vi "Read clEvtReportArray.vi"(8 "error in (no error)":errorcluster, 11 "VisualizeAppBase_class in":refnum<class "VisualizeAppBase_class.lvclass">) -> (0 "error out":errorcluster, 2 "clEvtReportArray":T1 {"Synx" format="%#_4g"}, 3 "VisualizeAppBase_class out":refnum<class "VisualizeAppBase_class.lvclass">)   [LabVIEW 2017, in "Visualization.lvlib" / "VisualizeAppBase_class.lvclass"]
uses:
  VisualizeAppBase_class.lvclass
  Modules/EventPlugins/EventPluginBaseClass/TypeDefs/clEvtReportArray.ctl
  Modules/EventPlugins/EventPluginBaseClass/TypeDefs/clEvtReport.ctl
  VisualizeAppBase_class.lvclass/VisualizeAppBase_class.ctl
  Modules/EventPlugins/EventPluginBaseClass/EventPluginBaseClass.lvclass
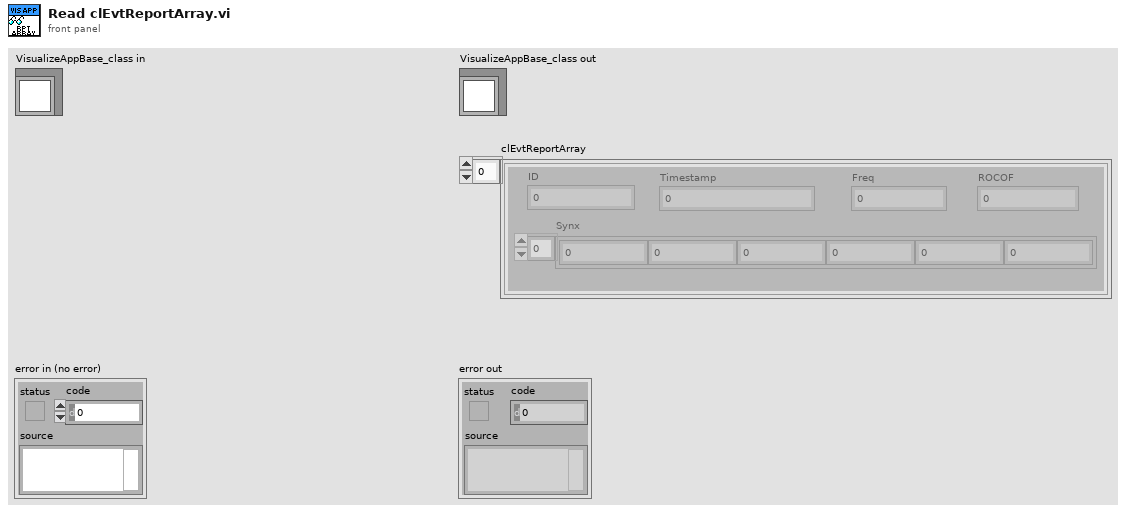
[diagram p1: front panel]
types:
  T1 = typedef "EventPlugins.lvlib/EventPluginBaseClass.lvclass/clEvtReportArray.ctl" = T2[]
  T2 = typedef "EventPlugins.lvlib/EventPluginBaseClass.lvclass/clEvtReport.ctl" = cluster{"Timestamp":dbl, "Synx":cdb[], "Freq":dbl, "ROCOF":dbl, "ID":i16}
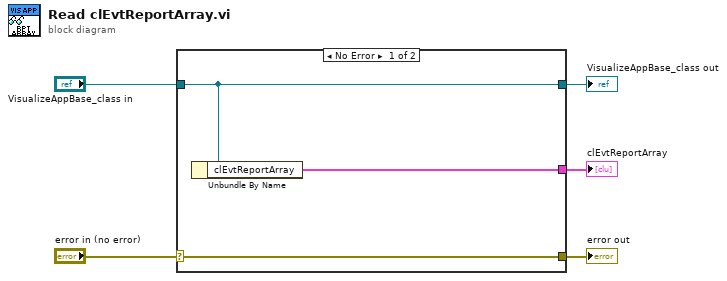
[diagram p0: block diagram]
diagram:
  n1 = case shown="No Error" "error in (no error)" {
    selector: "error in (no error)" -> [w8 w9]
    tunnel: [w8 w9] -> w4
    tunnel: [w7 w10] -> w2
    tunnel: "VisualizeAppBase_class in" -> [w7 w10]
    tunnel: [w6 _] -> w1
    frame No Error {
      n2 = Unbundle By Name(w7) -> ("clEvtReportArray"=w6:T1)
    }
    frame Error {
    }
  }
  "error out" <- w4
  "VisualizeAppBase_class out" <- w2
  "clEvtReportArray" <- w1
